vi "Get Name.vi"(8 "error in (no error)":errorcluster, 11 "Drive by Power in":refnum<class "Drive by Power.lvclass">) -> (0 "error out":errorcluster, 2 "Command Name":string, 3 "Drive by Power out":refnum<class "Drive by Power.lvclass">)   [LabVIEW 2014, in "Forward Drive.lvlib" / "Drive by Power.lvclass"]
uses:
  Drive by Power.lvclass
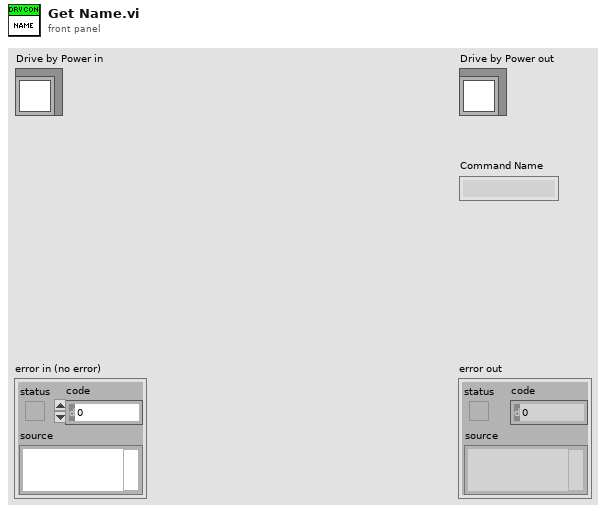
[diagram p1: front panel]
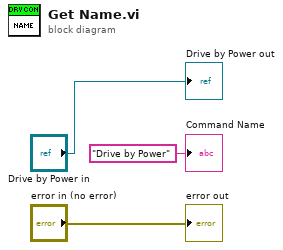
[diagram p0: block diagram]
diagram:
  "error out" <- "error in (no error)"
  "Drive by Power out" <- "Drive by Power in"
  "Command Name" <- "Drive by Power" ("Command Name")
